vi "T_rH.vi"(3 "HYTE -LOG":refnum<visa-resource-name>="COM8") -> (0 "Celsius":dbl, 1 "rH":dbl)   [LabVIEW 2019]
uses:
  <vilib>/Instr/_visa.llb/VISA Configure Serial Port (Instr).vi
panel:
  out "1":string
  out "2":string
  out "read buffer":string="5030148\rV021D1FFF\r$\r@\rI01010100B00725030"
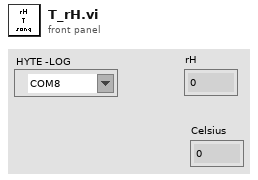
[diagram p1: front panel]
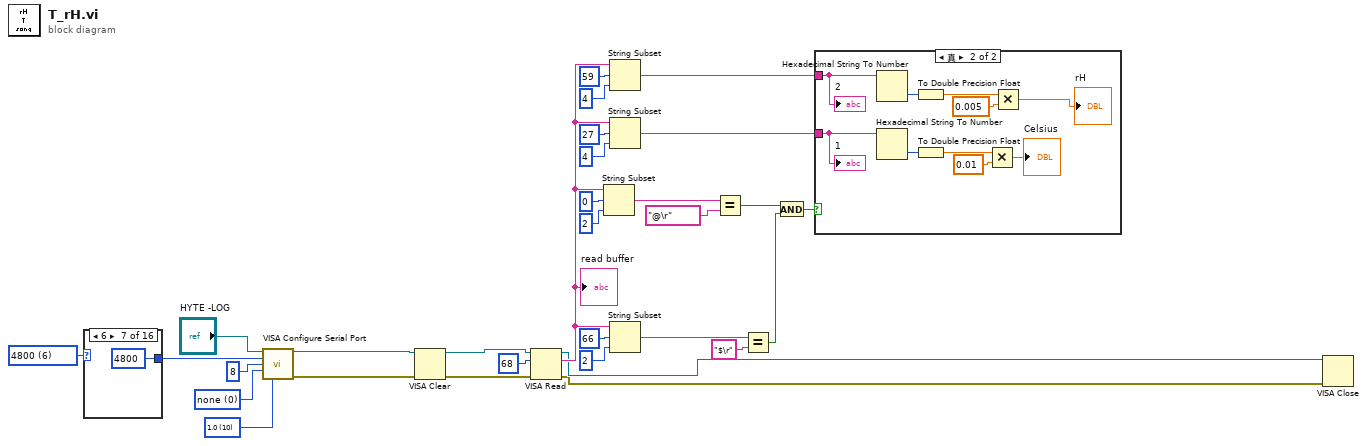
[diagram p0: block diagram]
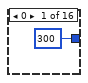
[diagram p3: hidden frame]
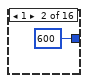
[diagram p4: hidden frame]
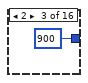
[diagram p5: hidden frame]
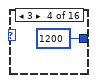
[diagram p6: hidden frame]
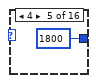
[diagram p7: hidden frame]
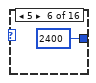
[diagram p8: hidden frame]
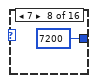
[diagram p9: hidden frame]
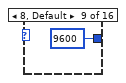
[diagram p10: hidden frame]
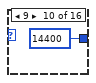
[diagram p11: hidden frame]
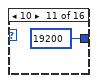
[diagram p12: hidden frame]
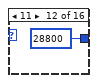
[diagram p13: hidden frame]
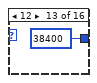
[diagram p14: hidden frame]
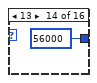
[diagram p15: hidden frame]
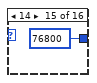
[diagram p16: hidden frame]
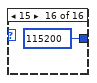
[diagram p17: hidden frame]
diagram:
  w28 = u16 6 items=["   300", "   600", "   900", "   1200", "   1800", "   2400", "   4800   ", "   7200", "   9600", "   14400", "   19200", "   28800", "   38400", "   56000", "   76800", "   115200"] ("buad rate：")
  w30 = u16 0 items=["none", "odd", "even"] ("parity：")
  w23 = u16 10 items=["1.0"=10, "1.5"=15, "2.0"=20] ("stop bits (10: 1 bit)")
  n1 = case shown="6" w28 {
    tunnel: [300 600 900 1200 1800 2400 4800 7200 9600 14400 19200 28800 38400 56000 76800 115200] -> w29
    frame 0 {
    }
    frame 1 {
    }
    frame 2 {
    }
    frame 3 {
    }
    frame 4 {
    }
    frame 5 {
    }
    frame 6 {
    }
    frame 7 {
    }
    frame 8, Default {
    }
    frame 9 {
    }
    frame 10 {
    }
    frame 11 {
    }
    frame 12 {
    }
    frame 13 {
    }
    frame 14 {
    }
    frame 15 {
    }
  }
  n2 = call-poly "VISA Configure Serial Port"("VISA resource name"="HYTE -LOG", "baud rate (9600)"=w29, "data bits (8)"=u16 8, "parity (0:none)"=w30, "stop bits (10: 1 bit)"=w23) -> ("VISA resource name out"=w27:refnum<visa-resource-name>, "error out"=w26:errorcluster)  [unwired: 9 in]
  n3 = VISA Clear(VISA resource name=w27, error in (no error)=w26) -> (VISA resource name out=w25:refnum<visa-resource-name>, error out=w24:errorcluster)
  n4 = VISA Read(VISA resource name=w25, byte count=u32 68, error in (no error)=w24) -> (VISA resource name out=w2:refnum<visa-resource-name>, read buffer=w3:string, error out=w1:errorcluster)  [unwired: 1 out]
  "read buffer" <- w3
  n5 = String Subset(string=w3, offset (0)=0 ("偏移量(0)"), length (rest)=2 ("长度（剩余）")) -> (substring=w14:string)
  n6 = String Subset(string=w3, offset (0)=59 ("偏移量(0)"), length (rest)=4 ("长度（剩余）")) -> (substring=w20:string)
  n7 = String Subset(string=w3, offset (0)=27 ("偏移量(0)"), length (rest)=4 ("长度（剩余）")) -> (substring=w19:string)
  n8 = String Subset(string=w3, offset (0)=66 ("偏移量(0)"), length (rest)=2 ("长度（剩余）")) -> (substring=w15:string)
  n9 = Equal?(x=w14, y="@\r") -> (x = y?=w16:bool)
  n10 = Equal?(x=w15, y="$\r") -> (x = y?=w17:bool)
  n11 = And(x=w16, y=w17) -> (x .and. y?=w18:bool)
  n12 = case shown="真" w18 {
    tunnel: w19 -> [_ w57]
    tunnel: w20 -> [_ w56]
    frame False {
    }
    frame True {
      n13 = Hexadecimal String To Number(string=w56) -> (number=w52:u32)  [unwired: 2 in, 1 out]
      n14 = Hexadecimal String To Number(string=w57) -> (number=w55:u32)  [unwired: 2 in, 1 out]
      n15 = To Double Precision Float(number=w52) -> (double precision float=w51:dbl)
      n16 = To Double Precision Float(number=w55) -> (double precision float=w54:dbl)
      n17 = Multiply(x=w54, y=0.01) -> (x*y=→"Celsius":dbl)
      n18 = Multiply(x=w51, y=0.005) -> (x*y=→"rH":dbl)
      "1" <- w57
      "2" <- w56
    }
  }
  n19 = VISA Close(VISA resource name=w2, error in (no error)=w1) -> ()  [unwired: 1 out]
